vi "Wrapper.vi"(0 "Controller in":refnum<class "Controller.lvclass">, 1 "Data":refnum<class "Data.lvclass">, 2 "ID":string, 5 "error in":errorcluster) -> (14 "Controller out":refnum<class "Controller.lvclass">, 19 "error out":errorcluster)   [LabVIEW 2014, in "Controller.lvlib" / "Update Data MSG.lvclass"]
uses:
  Update Data MSG.lvclass
  Controller.lvclass
  reusable/Data/Data.lvclass
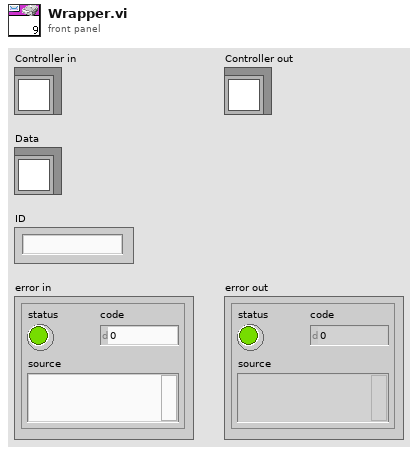
[diagram p1: front panel]
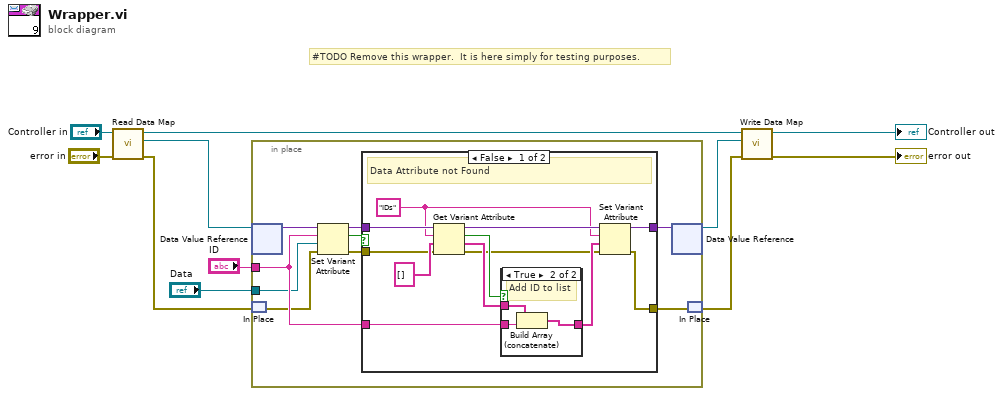
[diagram p0: block diagram]
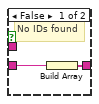
[diagram p2: hidden frame]
diagram:
  # "#TODO Remove this wrapper.  It is here simply for testing purposes."
  n1 = call "Read Data Map.vi"("error in"="error in", "Controller in"="Controller in") -> ("error out"=w2:errorcluster, "MAP DVR"=w4:refnum<data-value>, "Controller out"=w7:refnum<class "Controller.lvclass">)  [unwired: 7 in]
  n2 = in-place {
    in-place-border: "ID" -> [w20]
    in-place-border: "Data" -> [w17]
    n3 = in-place-dvr #1(w4) -> (w16:variant)  [unwired: 1 out]
    n4 = in-place-match #2(w2) -> (w13:errorcluster)
    n5 = Set Variant Attribute(Variant=w16, name=w20, value=w17, error in=w13) -> (Variant out=w19:variant, replaced=w18:bool, error out=w14:errorcluster)
    n6 = case shown="False" w18 {
      tunnel: w19 -> [w32 w39]
      tunnel: w20 -> [w26 _]
      tunnel: [w24 w39] -> w15
      tunnel: w14 -> [w23 w38]
      tunnel: [w21 w38] -> w12
      frame False {
        w29 = "IDs" ("name")
        # "Data Attribute not Found"
        n7 = Get Variant Attribute(Variant=w32, name=w29, default value (empty Variant)=string[] [], error in=w23) -> (duplicate Variant=w30:variant, found=w28:bool, value=w27:string[], error out=w22:errorcluster)
        n8 = case shown="True" w28 {
          tunnel: w27 -> [_ w37]
          tunnel: w26 -> [w34 w36]
          tunnel: [w33 w35] -> w25
          frame False {
            # "No IDs found"
            n9 = Build Array(w34) -> (w33:string[])
          }
          frame True {
            # "Add ID to list"
            n10 = Build Array (concatenate)(w37, w36) -> (w35:string[])
          }
        }
        n11 = Set Variant Attribute(Variant=w30, name=w29, value=w25, error in=w22) -> (Variant out=w24:variant, error out=w21:errorcluster)  [unwired: 1 out]
      }
      frame True {
        # "Data Attribute Found"
      }
    }
    n12 = in-place-dvr #1(w15) -> (w3:refnum<data-value>)  [unwired: 1 out]
    n13 = in-place-match #2(w12) -> (w1:errorcluster)
  }
  n14 = call "Write Data Map.vi"("error in"=w1, "MAP DVR"=w3, "Controller in"=w7) -> ("error out"=→"error out":errorcluster, "Controller out"=→"Controller out":refnum<class "Controller.lvclass">)  [unwired: 7 in]
